vi "Stop Core.vi"(10 "final error code":i32, 11 "IObserver in":refnum<class "IObserver.lvclass">) -> (3 "IObserver out":refnum<class "IObserver.lvclass">)   [LabVIEW 2020, in "MVA Framework.lvlib" / "IObserver.lvlib" / "IObserver.lvclass"]
doc: "(<B>Filename</B>: Actor Framework.lvlib:Actor.lvclass:Stop Core.vi)\n\nDefines what the actor does before it stops. Use the <B>final error code</B> input to determine whether the actor shut down in response to an error.\n\nBy default, this method does nothing. A descendant class may override it to define behavior, such as shutting down any processes the actor initiated in its override of the Actor Core method."
uses:
  IObserver.lvclass
  C:/Program Files/National Instruments/LabVIEW 2020/vi.lib/ActorFramework/Actor/Actor.lvclass
  composed-event-logger/Source/Composed Log/Types/Log Level.ctl
  IObserver.lvclass/IObserver.ctl
  composed-event-logger/Source/Composed Log/LoggerReference/LoggerReference.lvclass/LoggerReference.ctl
  composed-event-logger/Source/Composed Log/LoggerReference/Log Event.vi
  composed-event-logger/Source/Composed Log/LoggerReference/Log.vi
  composed-event-logger/Source/Composed Log/LoggerReference/Get Valid Event Time.vi
  composed-event-logger/Source/Composed Log/LoggerReference/Remove Stale Logs.vi
  <vilib>/Utility/LVClass/Get LV Class Name.vi
  <vilib>/ActorFramework/Actor/Actor.lvclass
  composed-event-logger/Source/Composed Log/Composed Log.lvlib
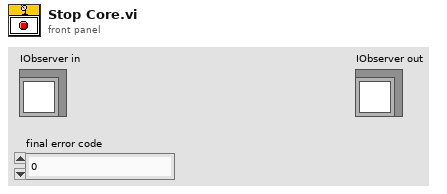
[diagram p1: front panel]
types:
  T1 = typedef "MVA Framework.lvlib/Composed Log.lvlib/Log Level.ctl" = enum16{"Debug", "Info", "Warning", "Error", "Critical"}
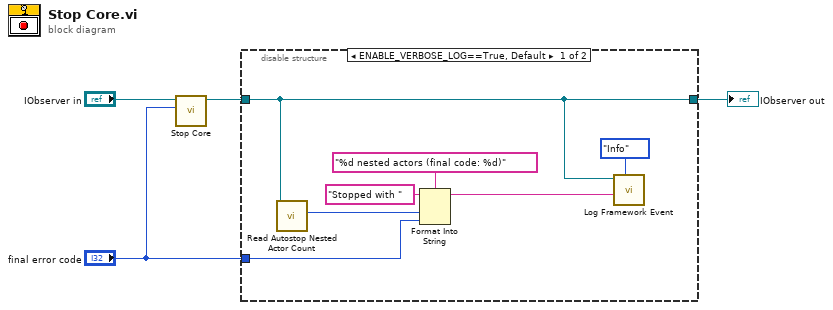
[diagram p0: block diagram]
diagram:
  n1 = call-parent "Stop Core.vi"("final error code"="final error code", "Actor in"="IObserver in") -> ("Actor out"=w2:refnum<class "IObserver.lvclass">)  [unwired: 9 in]
  n2 = disable-structure shown="ENABLE_VERBOSE_LOG==True, Default" {
    disable-tunnel: "final error code" -> [w5 _]
    disable-tunnel: w2 -> [w6 w12]
    disable-tunnel: [w6 w12] -> w1
    frame condition #0 (active) {
      # "Log stop events by default"
      n3 = call <vilib>:"Read Autostop Nested Actor Count.vi"("Actor in"=w6) -> ("Count"=w9:i32)  [unwired: 10 in]
      n4 = Format Into String(format string="%d nested actors (final code: %d)", initial string="Stopped with ", w9, w5) -> (resulting string=w8:string)  [unwired: 1 in, 1 out]
      n5 = call "Log Framework Event.vi"("Event Level (Debug)"=Log_Level."Info" ("Event Level"), "Data To Log"=w8, "IObserver in"=w6) -> ()  [unwired: 8 in, 1 out]
    }
    frame condition #1 {
      # "Remove all logging from this method at compile time"
    }
  }
  "IObserver out" <- w1
